vi "Error Case Test.vi"() -> ()   [LabVIEW 2019]
panel:
  in  "error code (0)":i32=63
  out "Boolean":bool
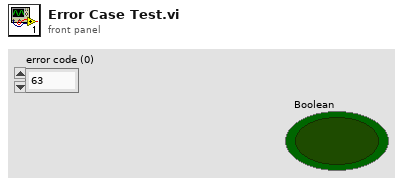
[diagram p1: front panel]
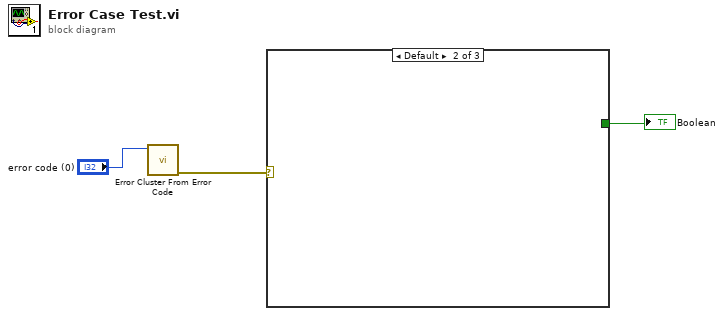
[diagram p0: block diagram]
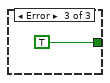
[diagram p3: hidden frame]
diagram:
  n1 = call <vilib>:"Error Cluster From Error Code.vi"("error code (0)"="error code (0)") -> ("error out"=w3:errorcluster)  [unwired: 8 in]
  n2 = case shown="Default" w3 {
    tunnel: [_ _ TRUE] -> w1
    frame No Error {
    }
    frame Default {
    }
    frame Error {
    }
  }
  "Boolean" <- w1
